vi "cleanDeviceType.vi"(0 "reference in":refnum<class "excelFile.lvclass">, 2 "device_type":string, 5 "error in (no error)":errorcluster) -> (14 "reference out":refnum<class "excelFile.lvclass">, 16 "deviceTypeCleaned":string, 19 "error out":errorcluster)   [LabVIEW 2016, in "excelFile.lvclass"]
uses:
  excelFile.lvclass
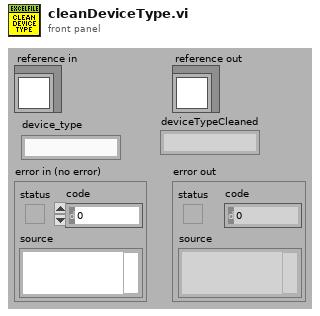
[diagram p1: front panel]
types:
  T1 = typedef "excelFile.lvclass/ObjectAttributesRef.ctl" = refnum<data-value>
  T2 = typedef "excelFile.lvclass/ObjectAttributes.ctl" = cluster{"MyAttribute":dbl, "path":string, "Refnum Excel":cluster{"Excel._Application":refnum<k7>, "Workbooks":refnum<k7>, "Open":refnum<k7>}, "data":string[][][], "save":bool, "fileType":T3, "rowsColor":u32[], "python_ref":refnum<class "python.lvclass">, "items_rows":i32[], "excel_range":i32[][], "TSR":cluster{"number":string, "TSR_path":path, "service_path":path, "email_to":string}, "excel_already_opened?":bool, "file_already_opened?":bool, "excel_protected_opened?":bool, "Refnum Cluster Worksheets":cluster{"Excel._Application":refnum<k7>, "Workbooks":refnum<k7>, "Open":refnum<k7>, "Worksheets":refnum<k7>, "Excel._Worksheet":refnum<k7>}, "#_rows_defective":i32, "#_rows_spare":i32}
  T3 = typedef "excelFile.lvclass/fileType.ctl" = enum16{"devices", "items", "partsTracking", "TSR"}
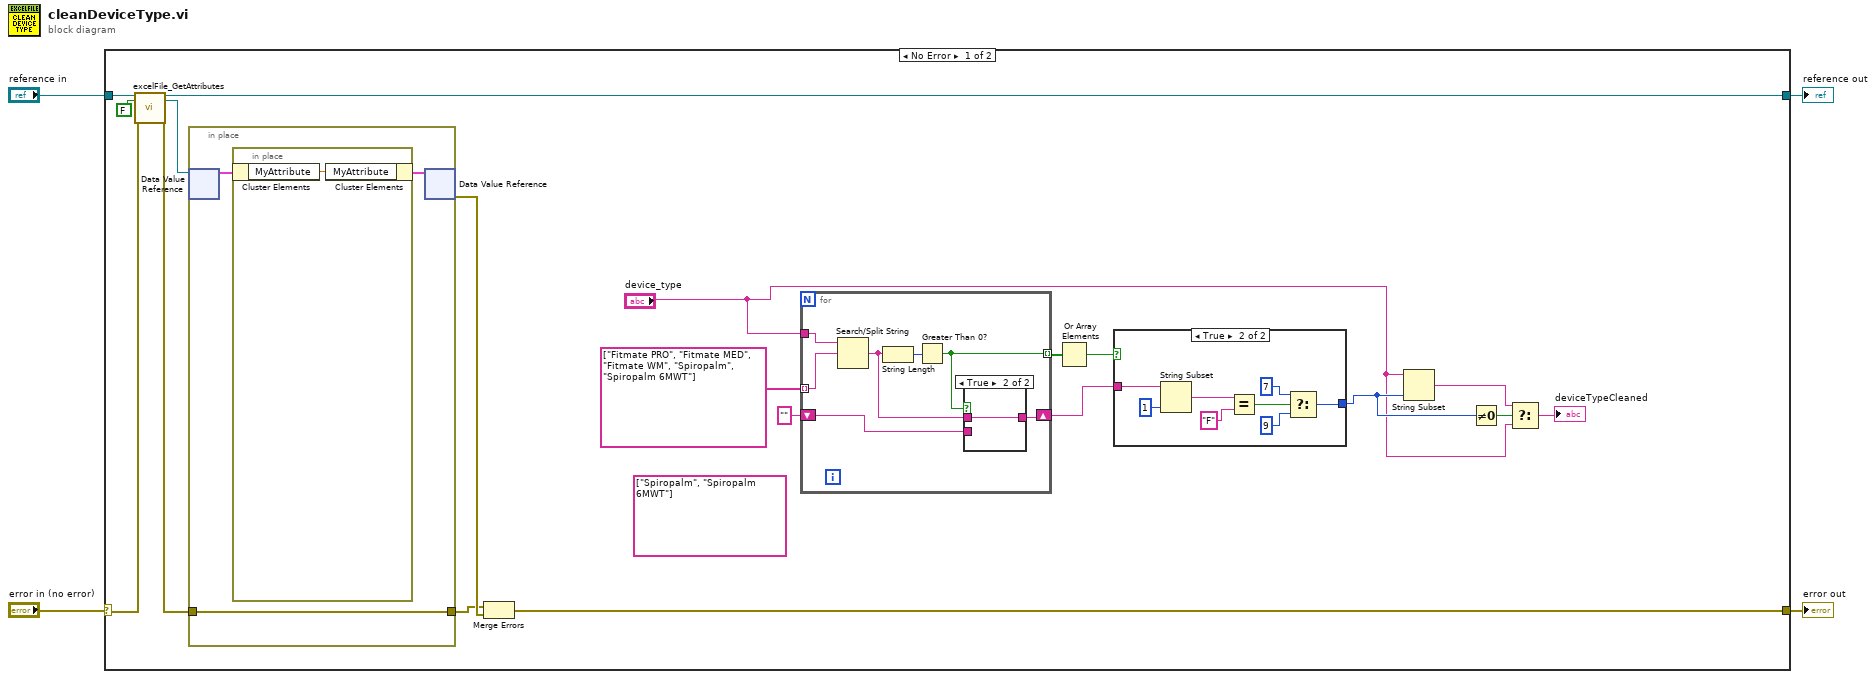
[diagram p0: block diagram]
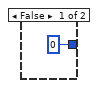
[diagram p2: hidden frame]
diagram:
  n1 = case shown="No Error" "error in (no error)" {
    selector: "error in (no error)" -> [w18 w47]
    tunnel: [w23 w47] -> w3
    tunnel: [w16 w46] -> w1
    tunnel: "reference in" -> [w20 w46]
    frame No Error {
      (unwired) string[] ["Spiropalm", "Spiropalm 6MWT"]
      n2 = call "excelFile_GetAttributes.vi"("reference in"=w20, "return data? (T)"=FALSE, "error in (no error)"=w18) -> ("reference out"=w16:refnum<class "excelFile.lvclass">, "attributes ref"=w15:T1, "error out"=w17:errorcluster)  [unwired: 13 in, 1 out]
      n3 = in-place {
        in-place-border: w17 -> [w42]
        in-place-border: [w42] -> w21
        n4 = in-place-dvr #1(w15) -> (w43:T2)  [unwired: 1 out]
        n5 = in-place {
          n6 = in-place-cluster #2(w43) -> ("MyAttribute"=w45:dbl)
          n7 = in-place-cluster #2("MyAttribute"=w45) -> (w44:T2)
        }
        n8 = in-place-dvr #1(w44) -> (w22:errorcluster)  [unwired: 1 out]
      }
      n9 = Merge Errors(w21, w22) -> (w23:errorcluster)
      n10 = for {
        tunnel: string[] ["Fitmate PRO", "Fitmate MED", "Fitmate WM", "Spiropalm", "Spiropalm 6MWT"] -> [w38] mode=indexing
        tunnel: "device_type" -> [w39]
        tunnel: [w36] -> w13 mode=indexing
        shift-right: [w34] -> w11
        shift-left: "" ("string") -> [w33]
        n11 = Search/Split String(string=w39, search string/char (-)=w38) -> (match + rest of string=w35:string)  [unwired: 1 in, 2 out]
        n12 = String Length(string=w35) -> (length=w37:i32)
        n13 = Greater Than 0?(x=w37) -> (x > 0?=w36:bool)
        n14 = case shown="True" w36 {
          tunnel: w35 -> [_ w41]
          tunnel: [w40 w41] -> w34
          tunnel: w33 -> [w40 _]
          frame False {
          }
          frame True {
          }
        }
      }
      n15 = Or Array Elements(Boolean array=w13) -> (logical OR=w12:bool)
      n16 = case shown="True" w12 {
        tunnel: w11 -> [_ w32]
        tunnel: [0 ("length (rest)") w25] -> w8
        frame False {
        }
        frame True {
          n17 = String Subset(string=w32, length (rest)=1 ("length (rest)")) -> (substring=w30:string)  [unwired: 1 in]
          n18 = Equal?(x=w30, y="F") -> (x = y?=w28:bool)
          n19 = Select(t=7 ("length (rest)"), s=w28, f=9 ("length (rest)")) -> (s? t:f=w25:i32)
        }
      }
      n20 = String Subset(string="device_type", length (rest)=w8) -> (substring=w7:string)  [unwired: 1 in]
      n21 = Not Equal To 0?(x=w8) -> (x != 0?=w9:bool)
      n22 = Select(t=w7, s=w9, f="device_type") -> (s? t:f=→"deviceTypeCleaned":string)
    }
    frame Error {
    }
  }
  "error out" <- w3
  "reference out" <- w1
